vi "dfd_Sym_FIR_Even_C.vi"() -> ()   [LabVIEW 2017, in "NI_DigFilterTemp.lvlib"]
uses:
  <vilib>/addons/Digital Filter Design/NI_DigFilterTemp.lvlib
panel:
  in  "String":string="\n\n/* ---- Constants ----*/\n#define %CapName%_N_TAPS %kTAPS%\n#define %CapName%_N_HALFTAPS ((%CapName%_N_TAPS+1)>>1)\n#define %CapName%_N_STATES %CapName%_N_TAPS\n\n/* ---- Global Variables Declaration ----*/\nstatic %CoefBType% %FilterBlkName%_Coef[%CapName%_N_HALFTAPS];\n%InternalFunctionsDeclaration%\n\n%ShiftDefine%\n\n%AssistantFunctions%\n\n/* ---- Implement the Fixed-Point Filter ---- */ \n%OutType% %FilterBlkName%_Filtering (%InType% sampleIn, %FilterBlkName%_State state)\n{\n\tI32 accA;\n\t%MultType% accB;\n\tint i, j;             \n\n\t/* Update the internal states */\n\tfor (i=(%CapName%_N_STATES-1); i>0; i--)\n\t\tstate[i] = state[i-1];\n\tstate[i] = (sampleIn << IN2DELAY);\n\n\t/* Filtering */\n\taccA = 0;\n\taccB = 0;\n\tfor (i=0, j=(%CapName%_N_TAPS-1); i < %CapName%_N_HALFTAPS; i++, j--)\n\t{\n\t\taccB = (%PreMultCast%state[i] << DELAY2MULT) + (%PreMultCast%state[j] << DELAY2MULT);\n\t\taccA += (%FilterBlkName%_%MultB%(accB, %FilterBlkName%_Coef[i]) << PROD2SUM);\n\t}\n\n\t%ApplyGainAccA%\n\n\treturn (%OutType%)accA;\n}\n\n/* ---- Internal Functions ---- */\n%InternalFunctions%\n\n/* ---- Filter Coefficients ---- */\nstatic %CoefBType% %FilterBlkName%_Coef[] = {\n%CoefficientsB%\n};\n"
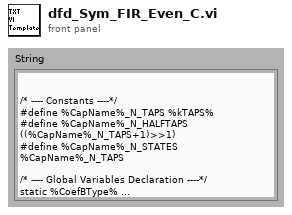
[diagram p1: front panel]
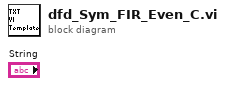
[diagram p0: block diagram]
diagram:
